vi "set_log_file_path.vi"(8 "error in (no error)":errorcluster, 11 "Path":path) -> (0 "error out":errorcluster)   [LabVIEW 2017, in "Vision.lvlib"]
uses:
  Vision.lvlib
  bin/Vision.dll
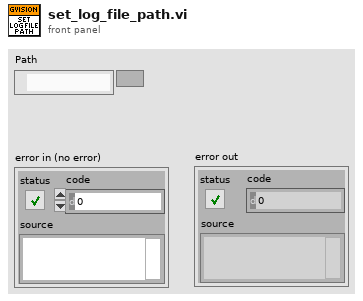
[diagram p1: front panel]
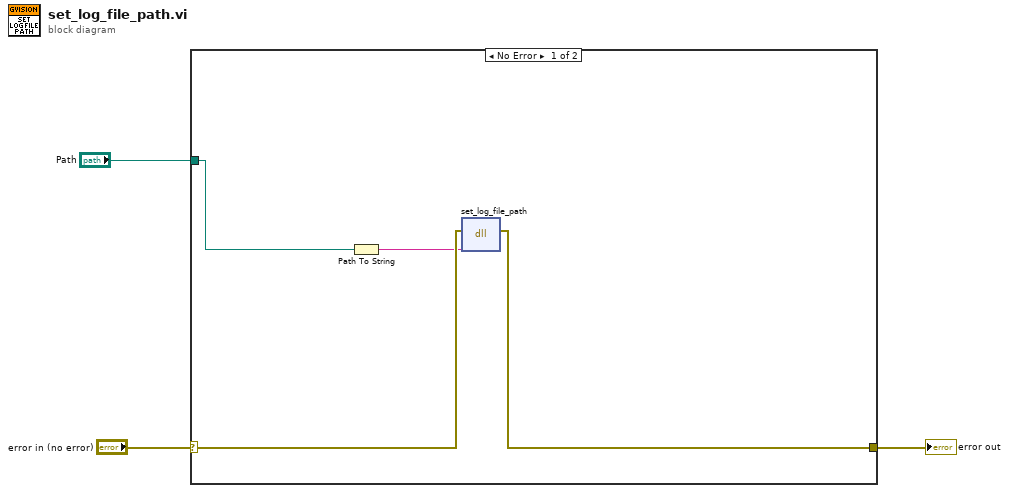
[diagram p0: block diagram]
diagram:
  n1 = case shown="No Error" "error in (no error)" {
    selector: "error in (no error)" -> [w7 w8]
    tunnel: [w4 w8] -> w2
    tunnel: "Path" -> [w6 _]
    frame No Error {
      n2 = Path To String(path=w6) -> (string=w5:string)
      n3 = dll-call lib="C:/Users/Caleb/Desktop/nebraska-silicon-lab/pixel-gantry-extra/LV/bin/Vision.dll" fn="set_log_file_path"(error in=w7, "new_log_file_path"=w5) -> (error out=w4:errorcluster)  [unwired: 4 in, 1 out]
    }
    frame Error {
    }
  }
  "error out" <- w2
